vi "GetJSONTextBlock.vi"(8 "error in (no error)":errorcluster, 10 "Block Start Offset":i32, 11 "String In":string) -> (0 "error out":errorcluster, 1 "Offset Past Block":i32, 2 "Matched Block Contents":string, 3 "String Out":string, 4 "Matched Block":string)   [LabVIEW 2013]
doc: "If the 'String In' character given by 'Block Start Offset' contains '{', '[', or '\"', 'Matched Block Contents' contains the contents of the block started by that character, respecting any nesting of braces or brackets. Otherwise, it contains the empty string.\n\nException: It skips initial whitespace before checking for the opening block characters above."
uses:
  <vilib>/Utility/error.llb/Error Cluster From Error Code.vi
  <vilib>/regexp/Match Regular Expression.xnode
  <vilib>/ErrorRing/Error Ring.xnode
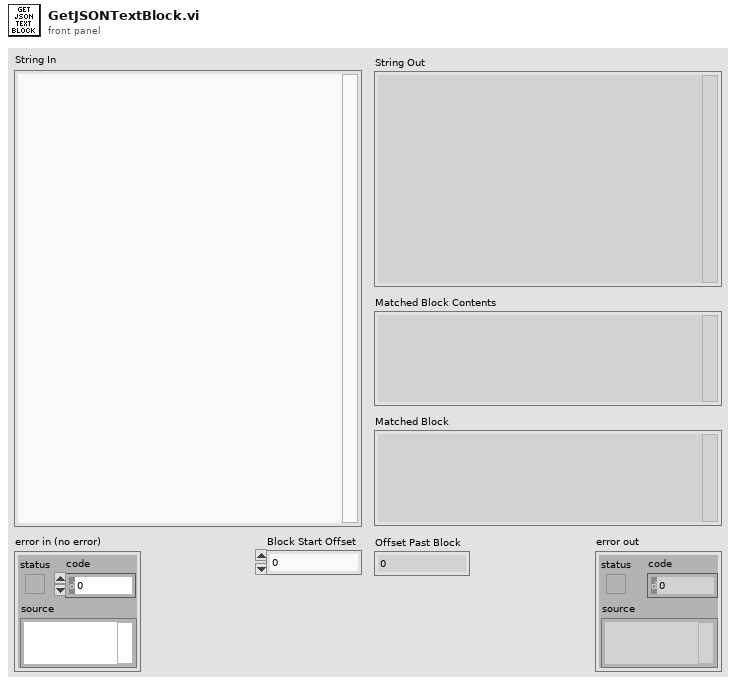
[diagram p1: front panel]
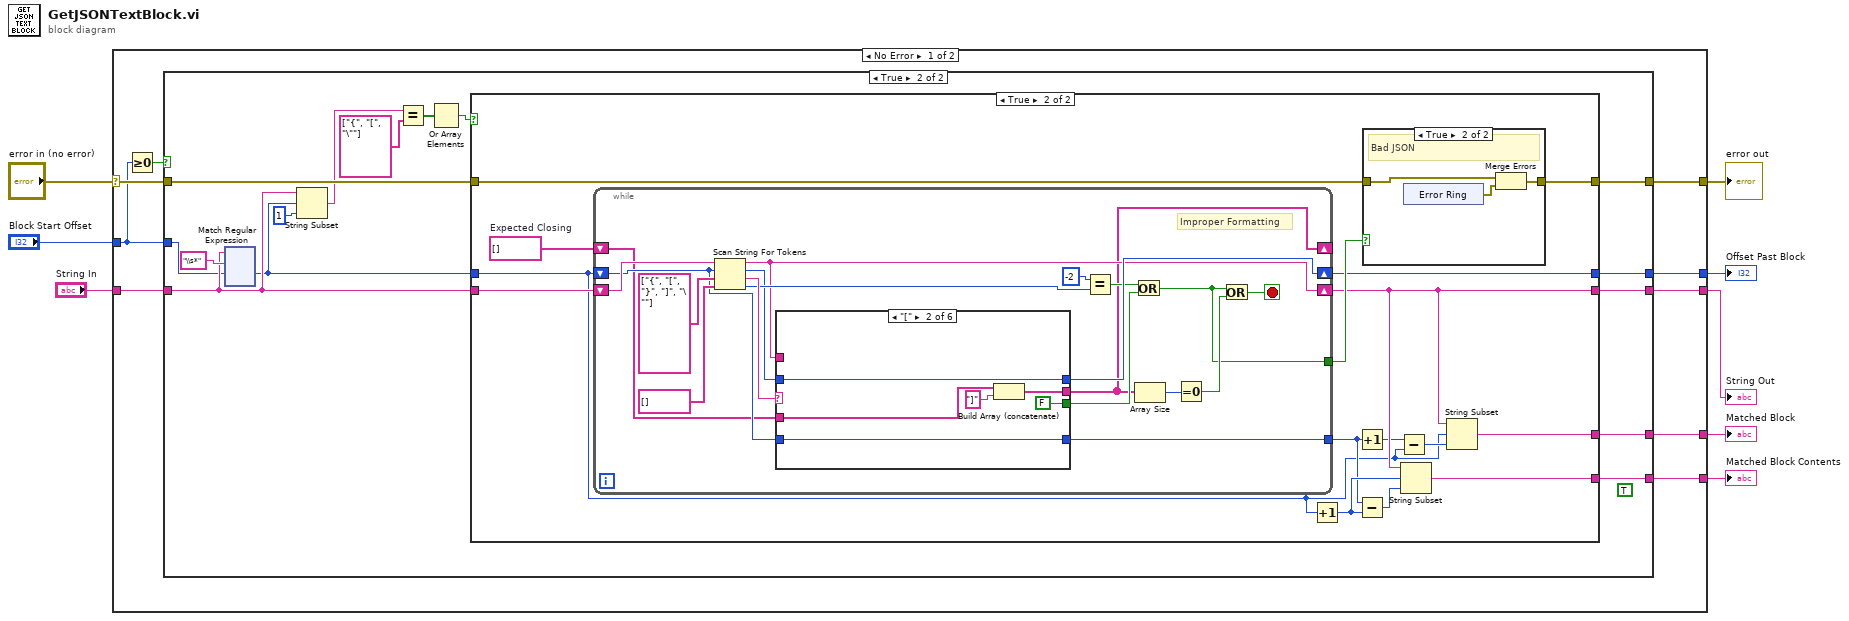
[diagram p0: block diagram]
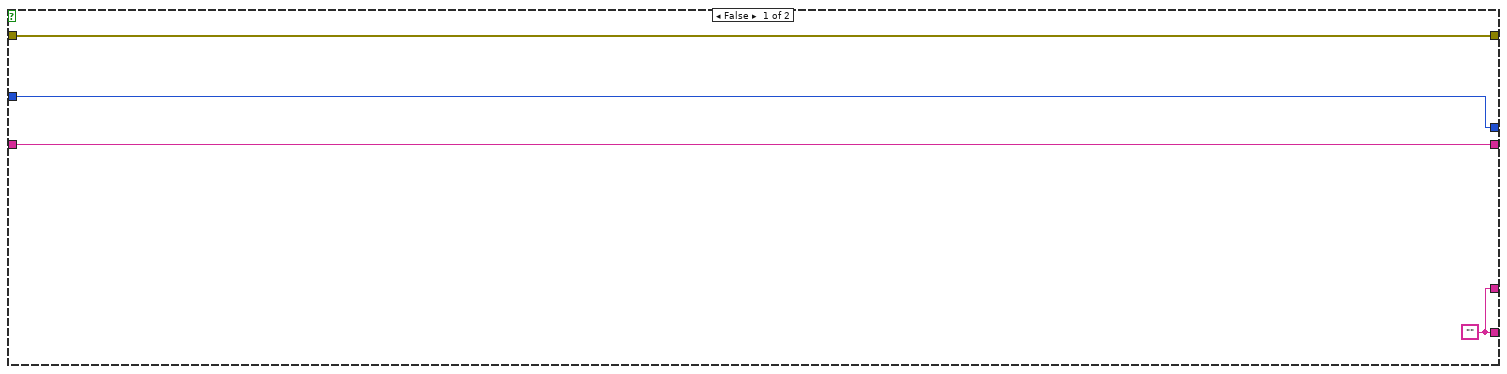
[diagram p2: hidden frame]
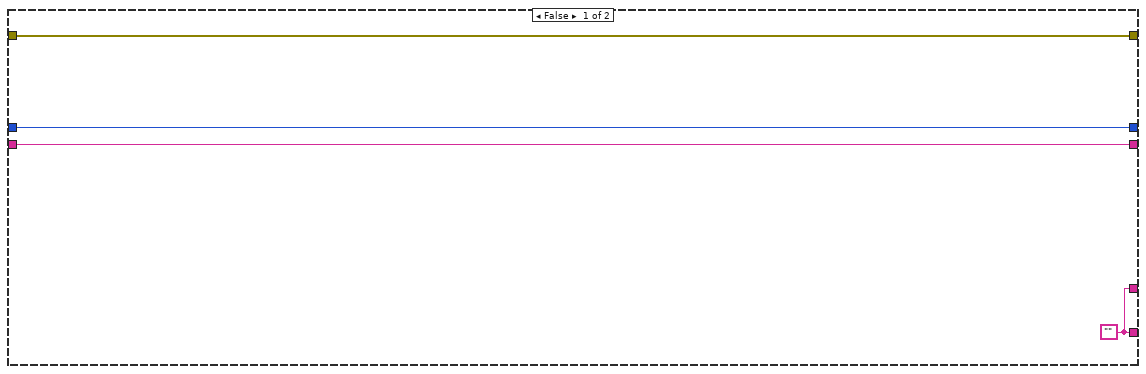
[diagram p3: hidden frame]
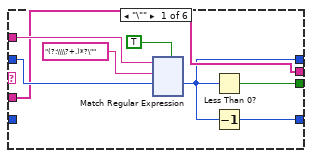
[diagram p5: hidden frame]
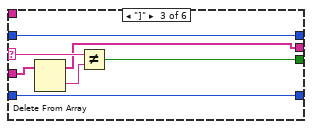
[diagram p6: hidden frame]
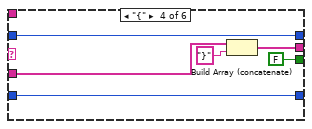
[diagram p7: hidden frame]
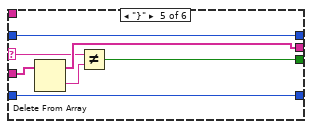
[diagram p8: hidden frame]
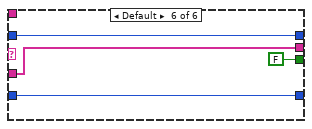
[diagram p9: hidden frame]
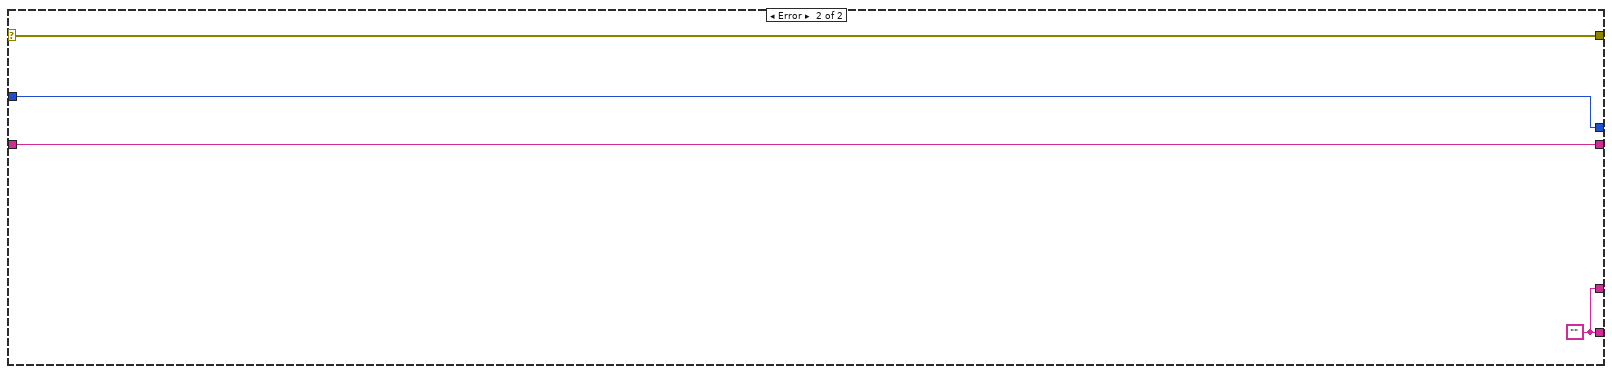
[diagram p10: hidden frame]
diagram:
  n1 = case shown="No Error" "error in (no error)" {
    selector: "error in (no error)" -> [w16 w352]
    tunnel: [w17 w352] -> w7
    tunnel: "String In" -> [w12 w351]
    tunnel: [w15 w351] -> w5
    tunnel: [w14 w349] -> w4
    tunnel: [w13 w350] -> w3
    tunnel: "Block Start Offset" -> [w9 w350]
    tunnel: [w11 w349] -> w1
    frame No Error {
      n2 = Greater Or Equal To 0?(x=w9) -> (x >= 0?=w10:bool)
      n3 = case shown="True" w10 {
        tunnel: [w21 w36] -> w17
        tunnel: w16 -> [w21 w35]
        tunnel: [w19 w34] -> w15
        tunnel: [w18 w33] -> w14
        tunnel: [w20 w32] -> w13
        tunnel: w9 -> [w20 w23]
        tunnel: w12 -> [w19 w24]
        tunnel: [w18 w26] -> w11
        frame False {
          w18 = ""
        }
        frame True {
          (unwired) TRUE ("multiline? (F)")
          n4 = xnode "Match Regular Expression"("input string"=w24, "regular expression"="\\s*", "offset (0)"=w23) -> ("offset past match"=w22:i32)  [unwired: 3 in, 4 out]
          n5 = String Subset(string=w24, offset (0)=w22, length (rest)=1 ("length (rest)")) -> (substring=w31:string)
          n6 = Equal?(x=w31, y=string[] ["{", "[", "\""] ("operators (none)")) -> (x = y?=w29:bool[])
          n7 = Or Array Elements(Boolean array=w29) -> (logical OR=w28:bool)
          n8 = case shown="True" w28 {
            tunnel: [w153 w165] -> w36
            tunnel: w35 -> [w153 w164]
            tunnel: [w152 w162] -> w34
            tunnel: [w151 w163] -> w33
            tunnel: [w154 w160] -> w32
            tunnel: w22 -> [w154 w155]
            tunnel: w24 -> [w152 w156]
            tunnel: [w151 w161] -> w26
            frame False {
              w151 = ""
            }
            frame True {
              w167 = string[] []  # Expected Closing
              n9 = while {
                shift-right: [w188] -> w160
                shift-left: w155 -> [w186]
                shift-right: [w187] -> w162
                shift-left: w156 -> [w194]
                tunnel: [w185] -> w158
                shift-right: [w179] -> _
                shift-left: w167 -> [w183]
                tunnel: [w178] -> w166
                stop <- w190 stop-if-true
                # "Improper Formatting"
                n10 = Scan String For Tokens(6:string[] [] ("delimiters (\\s,\\t,\\r,\\n)"), 7:string[] ["{", "[", "}", "]", "\""] ("operators (none)"), 8:w186, 9:w194) -> (0:w192:i32, 1:w193:string, 2:w189:i32, 3:w187:string)  [unwired: 2 in]
                n11 = case shown="\"[\"" w193 {
                  selector: w193 -> [_ _ w328 _ w340 _]
                  tunnel: [w198 w324 w331 w337 w344 w348] -> w188
                  tunnel: w189 -> [w203 w324 w331 w337 w344 w348]
                  tunnel: w187 -> [w202 _ _ _ _ _]
                  tunnel: w186 -> [_ w323 w330 w336 w343 w347]
                  tunnel: [w200 w323 w330 w336 w343 w347] -> w185
                  tunnel: w183 -> [w199 w321 w325 w335 w342 w345]
                  tunnel: [w199 w320 w326 w334 w341 w345] -> w179
                  tunnel: [w197 FALSE w329 FALSE w338 FALSE] -> w180
                  frame "\"" {
                    n12 = xnode "Match Regular Expression"("input string"=w202, "regular expression"="(?:\\\\?+.)*?\"", "offset (0)"=w203, "multiline? (F)"=TRUE) -> ("offset past match"=w198:i32)  [unwired: 2 in, 4 out]
                    n13 = Less Than 0?(x=w198) -> (x < 0?=w197:bool)
                    n14 = Decrement(x=w198) -> (x-1=w200:i32)
                  }
                  frame "[" {
                    n15 = Build Array (concatenate)(w321, "]") -> (w320:string[])
                  }
                  frame "]" {
                    n16 = Delete From Array(array=w325) -> (deleted portion=w327:string, array with subset deleted=w326:string[])  [unwired: 2 in]
                    n17 = Not Equal?(x=w328, y=w327) -> (x != y?=w329:bool)
                  }
                  frame "{" {
                    n18 = Build Array (concatenate)(w335, "}") -> (w334:string[])
                  }
                  frame "}" {
                    n19 = Delete From Array(array=w342) -> (deleted portion=w339:string, array with subset deleted=w341:string[])  [unwired: 2 in]
                    n20 = Not Equal?(x=w340, y=w339) -> (x != y?=w338:bool)
                  }
                  frame Default {
                  }
                }
                n21 = Equal?(x=-2, y=w192) -> (x = y?=w184:bool)
                n22 = Or(x=w184, y=w180) -> (x .or. y?=w178:bool)
                n23 = Array Size(array=w179) -> (size(s)=w181:i32)
                n24 = Equal To 0?(x=w181) -> (x = 0?=w182:bool)
                n25 = Or(x=w178, y=w182) -> (x .or. y?=w190:bool)
              }
              n26 = Increment(x=w155) -> (x+1=w168:i32)
              n27 = Increment(x=w158) -> (x+1=w159:i32)
              n28 = Subtract(x=w158, y=w168) -> (x-y=w169:i32)
              n29 = case shown="True" w166 {
                tunnel: [w170 w171] -> w165
                tunnel: w164 -> [w170 w173]
                frame False {
                }
                frame True {
                  # "Bad JSON"
                  n30 = xnode "Error Ring"() -> ("error out"=w172:errorcluster)
                  n31 = Merge Errors(w173, w172) -> (w171:errorcluster)
                }
              }
              n32 = Subtract(x=w159, y=w155) -> (x-y=w157:i32)
              n33 = String Subset(string=w162, offset (0)=w168, length (rest)=w169) -> (substring=w163:string)
              n34 = String Subset(string=w162, offset (0)=w155, length (rest)=w157) -> (substring=w161:string)
            }
          }
        }
      }
    }
    frame Error {
      w349 = ""
    }
  }
  "error out" <- w7
  "String Out" <- w5
  "Matched Block Contents" <- w4
  "Offset Past Block" <- w3
  "Matched Block" <- w1
